vi "WriteDoubleGlobals.vi"(0 "controller in":refnum<k24>, 7 "variable number":i32, 9 "values":dbl[](array[numeric]), 11 "error in (no error)":errorcluster) -> (4 "controller out":refnum<k24>, 15 "error out":errorcluster)   [LabVIEW 2019]
uses:
  C:/Users/patrick/Documents/GitHub/Aerotech-Delay-Line/lvsrc/Aerotech-Ensemble-LabVIEW/2010-5.6/Bin/Aerotech.Ensemble.dll
  Bin/Aerotech.Ensemble.dll
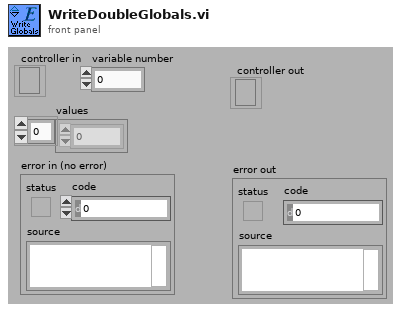
[diagram p1: front panel]
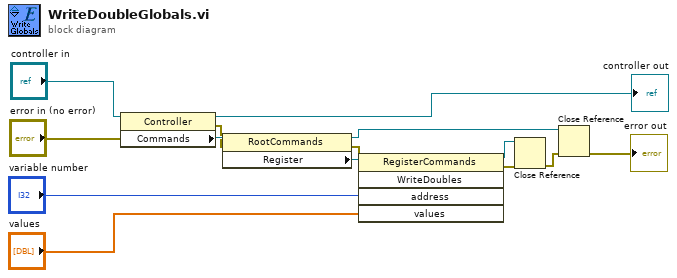
[diagram p0: block diagram]
diagram:
  n1 = property class="Controller"(reference="controller in", error in="error in (no error)") -> (reference out=→"controller out":refnum<k24>, error out=w11:errorcluster, "Commands"=w12:refnum<k24>)
  n2 = property class="RootCommands"(reference=w12, error in=w11) -> (reference out=w5:refnum<k24>, error out=w9:errorcluster, "Register"=w10:refnum<k24>)
  n3 = invoke class="RegisterCommands" method="WriteDoubles"(reference=w10, error in=w9, "address"="variable number", "values"="values") -> (reference out=w7:refnum<k24>, error out=w8:errorcluster)  [unwired: 1 in, 3 out]
  n4 = Close Reference(reference=w7, error in (no error)=w8) -> (error out=w6:errorcluster)
  n5 = Close Reference(reference=w5, error in (no error)=w6) -> (error out=→"error out":errorcluster)
